vi "searchEditDevice.vi"(8 "error in (no error)":errorcluster, 11 "reference in":refnum<class "Project Panels.lvclass">=refnum) -> (0 "error out":errorcluster, 2 "saved?":bool, 3 "reference out":refnum<class "Project Panels.lvclass">)   [LabVIEW 2014, in "Project Panels.lvclass"]
uses:
  Project Panels.lvclass
  SYS/Devices Controller_llb/deviceType.ctl
  deviceState.ctl
  SYS/Devices Controller_llb/Devices Controller.lvclass
panel:
  in  "Stop Button":bool
  out "Status bar":string="Fill in the control and press Sarch Item button....."
  in  "Search Item":bool
  in  "S/N:":string
  in  "Device Type:":T1=enum."k4b2"
  out "title":string="Searching Item Panel"
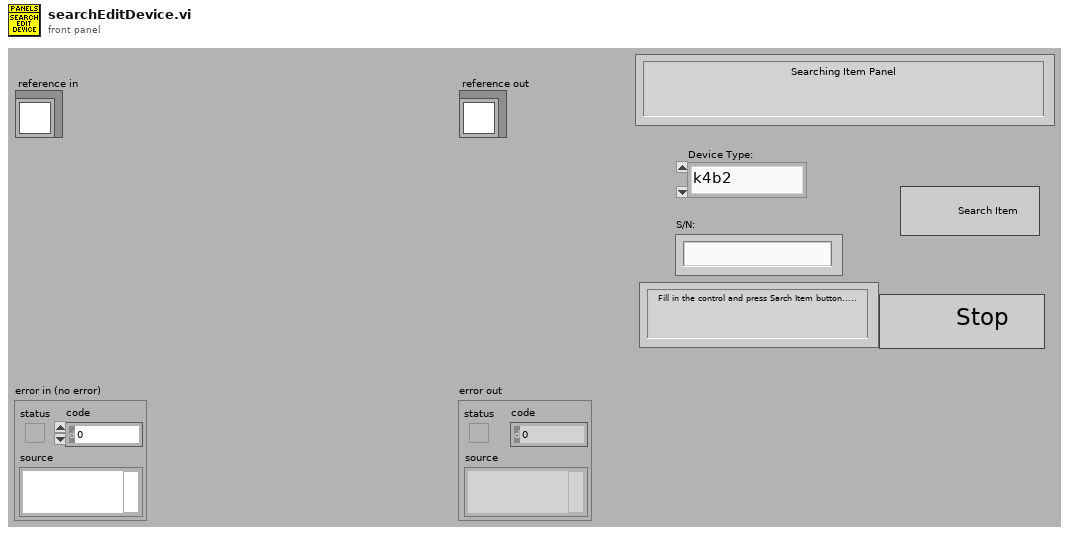
[diagram p1: front panel]
types:
  T1 = typedef "Devices Controller.lvclass/deviceType.ctl" = enum16{"k5", "k4b2", "fitmate", "cpet", "rmr", "bodyBoxPft", "bp", "pp"}
  T2 = typedef "Project Panels.lvclass/deviceState.ctl" = enum16{"check", "initiate", "waitEvent", "dataFromPDF", "getDetails", "save", "close", "stop"}
  T3 = typedef "Project Panels.lvclass/ObjectAttributesRef.ctl" = refnum<data-value>
  T4 = typedef "Project Panels.lvclass/ObjectAttributes.ctl" = cluster{"MyAttribute":dbl, "device_controller_ref":refnum<class "Devices Controller.lvclass">, "file_controller_ref":refnum<class "File Controller.lvclass">, "item_controller_ref":refnum<class "Items Controller.lvclass">, "item_tables":cluster{"checkIN":string[][], "checkOUT":string[][], "storage":string[][]}, "quickbook_table":cluster{"notes":string[][]}, "notification_controller_ref":refnum<class "Notification Controller.lvclass">, "partstracking_controller_ref":refnum<class "PartsTracking Controller.lvclass">, "product_tables":cluster{"k4b2":string[][], "fitmate":string[][], "RMR":string[][], "CPET":string[][], "BP":string[][], "PP":string[][], "k5":string[][], "bb-pft":string[][]}, "rowsColour":u32[]}
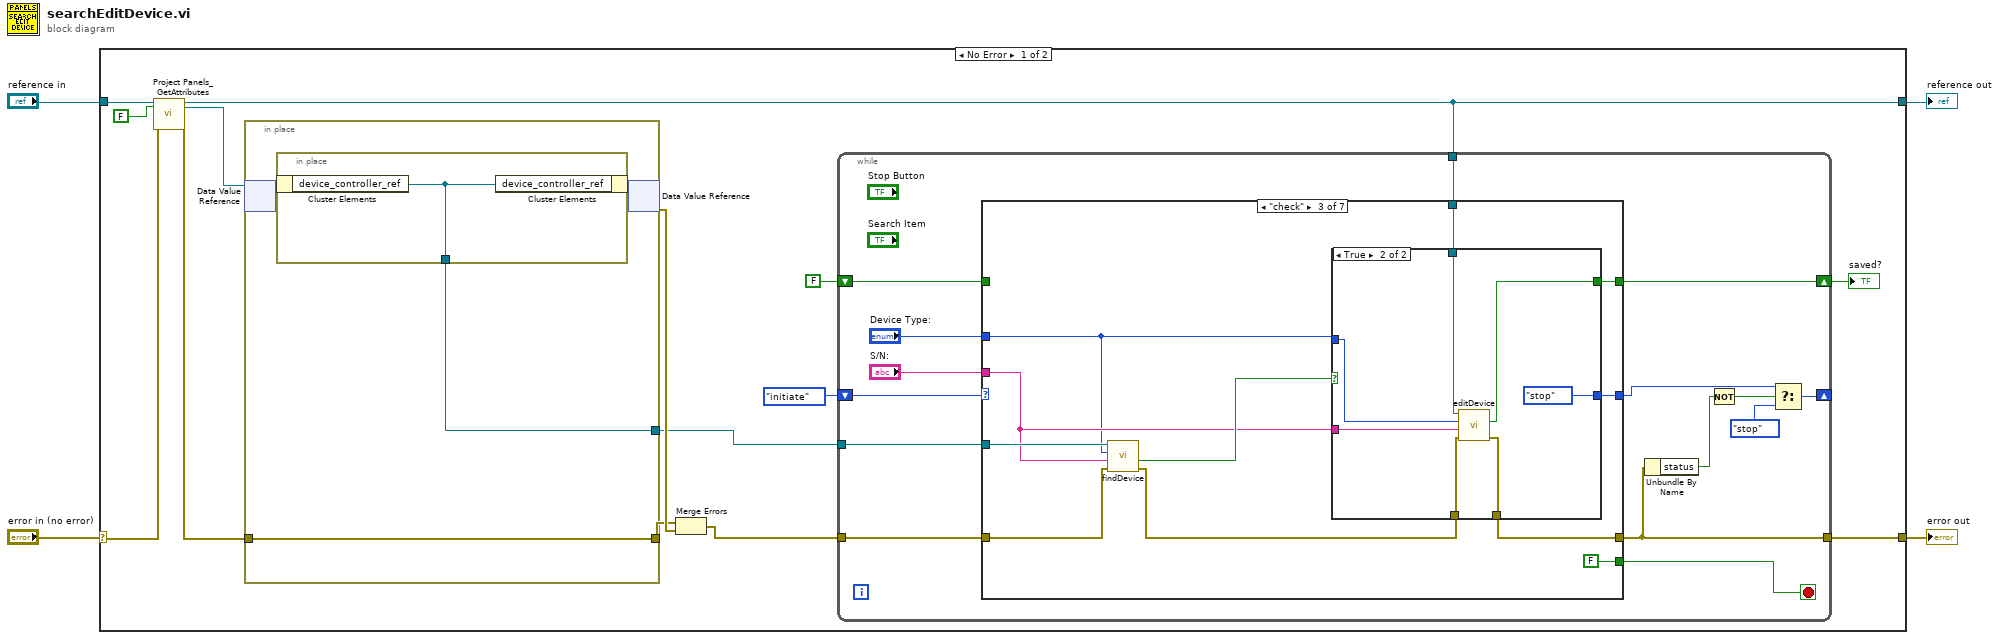
[diagram p0: block diagram]
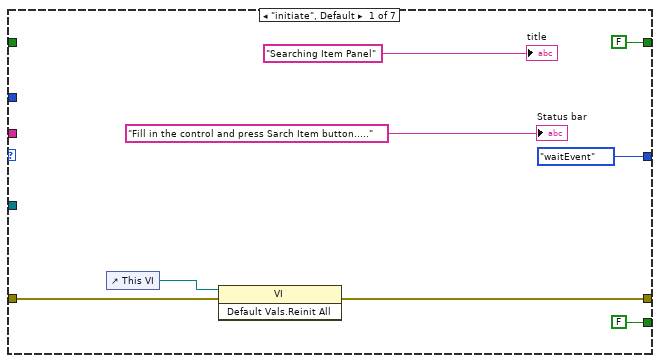
[diagram p2: hidden frame]
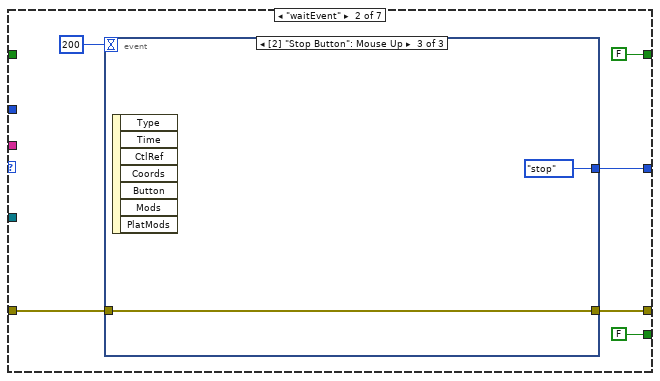
[diagram p3: hidden frame]
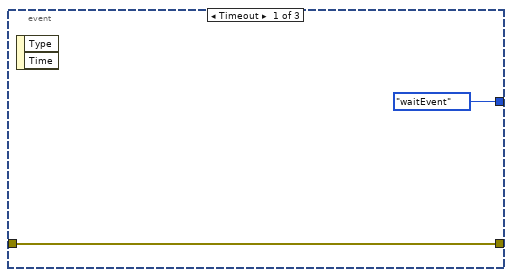
[diagram p4: hidden frame]
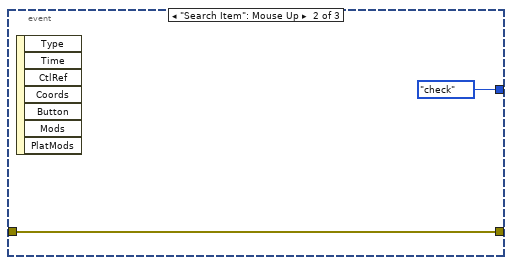
[diagram p5: hidden frame]
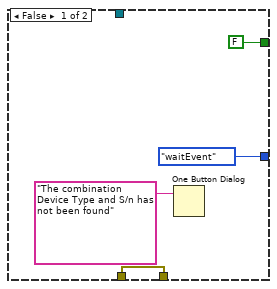
[diagram p6: hidden frame]
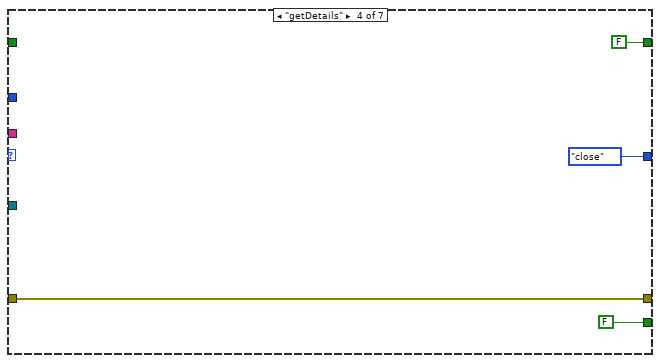
[diagram p7: hidden frame]
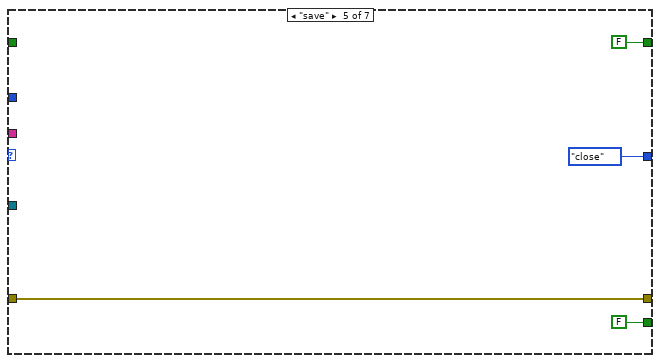
[diagram p8: hidden frame]
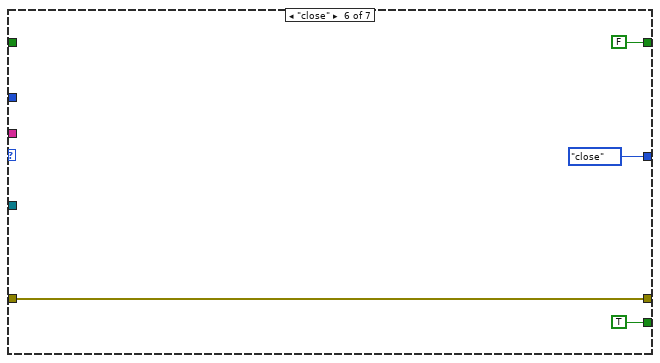
[diagram p9: hidden frame]
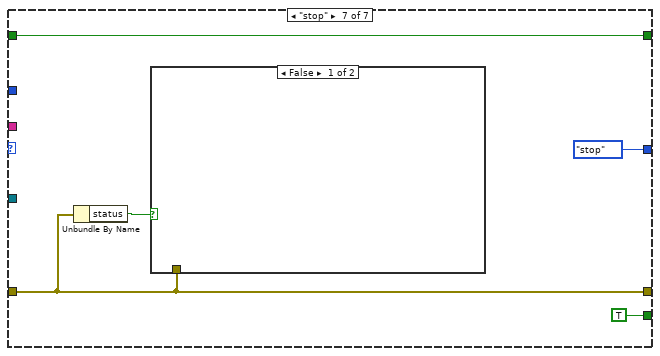
[diagram p10: hidden frame]
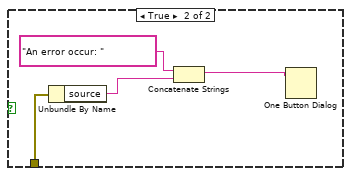
[diagram p11: hidden frame]
diagram:
  n1 = case shown="No Error" "error in (no error)" {
    selector: "error in (no error)" -> [w14 w103]
    tunnel: [w11 w103] -> w3
    tunnel: [w9 w102] -> w1
    tunnel: "reference in" -> [w16 w102]
    frame No Error {
      n2 = call "Project Panels_GetAttributes.vi"("reference in"=w16, "return data? (T)"=FALSE, "error in (no error)"=w14) -> ("reference out"=w9:refnum<class "Project Panels.lvclass">, "attributes ref"=w12:T3, "error out"=w13:errorcluster)  [unwired: 13 in, 1 out]
      n3 = in-place {
        in-place-border: w13 -> [w98]
        in-place-border: [w98] -> w17
        in-place-border: [w97] -> w5
        n4 = in-place-dvr #1(w12) -> (w99:T4)  [unwired: 1 out]
        n5 = in-place {
          in-place-border: [w101] -> w97
          n6 = in-place-cluster #2(w99) -> ("device_controller_ref"=w101:refnum<class "Devices Controller.lvclass">)
          n7 = in-place-cluster #2("device_controller_ref"=w101) -> (w100:T4)
        }
        n8 = in-place-dvr #1(w100) -> (w18:errorcluster)  [unwired: 1 out]
      }
      n9 = Merge Errors(w17, w18) -> (w6:errorcluster)
      n10 = while {
        tunnel: w6 -> [w33]
        tunnel: [w29] -> w11
        shift-right: [w30] -> _
        shift-left: deviceState."initiate" ("state") -> [w32]
        tunnel: w9 -> [w23]
        shift-right: [w21] -> w8
        shift-left: FALSE ("saved?") -> [w20]
        tunnel: w5 -> [w19]
        stop <- w22 stop-if-true
        n11 = case shown="\"check\"" w32 {
          tunnel: w33 -> [w35 w47 w59 w78 w82 w86 w89]
          tunnel: [w34 w46 w62 w78 w82 w86 w89] -> w29
          tunnel: [deviceState."waitEvent" ("state") w44 w64 deviceState."close" ("f") deviceState."close" ("f") deviceState."close" ("f") deviceState."stop" ("f")] -> w31
          tunnel: "Device Type:" -> [_ _ w54 _ _ _ _]
          tunnel: "S/N:" -> [_ _ w55 _ _ _ _]
          tunnel: w23 -> [_ _ w63 _ _ _ _]
          tunnel: [FALSE FALSE FALSE FALSE FALSE TRUE TRUE] -> w22
          tunnel: [FALSE ("saved?") FALSE ("saved?") w60 FALSE ("saved?") FALSE ("saved?") FALSE ("saved?") w88] -> w21
          tunnel: w20 -> [_ _ _ _ _ _ w88]
          tunnel: w19 -> [_ _ w57 _ _ _ _]
          frame "initiate", Default {
            n12 = control-ref of="This VI"() -> (w36:refnum<vi>)
            n13 = invoke class="VI" method="Default Vals.Reinit All"(reference=w36, error in=w35) -> (error out=w34:errorcluster)  [unwired: 1 in, 2 out]
            "title" <- "Searching Item Panel" ("title")
            "Status bar" <- "Fill in the control and press Sarch Item button....." ("Status bar")
          }
          frame "waitEvent" {
            n14 = event shown="[2] \"Stop Button\": Mouse Up" {
              selector: _ -> [_ _ _]
              dyn-events: _ -> [_ _ _]
              timeout: 200 -> [_ _ _]
              tunnel: w47 -> [w49 w51 w52]
              tunnel: [w49 w51 w52] -> w46
              tunnel: [deviceState."waitEvent" ("f") deviceState."check" ("f") deviceState."stop" ("f")] -> w44
              event Timeout {
                n15 = event-data() -> ()  [unwired: 1 in, 2 out]
              }
              event "Search Item": Mouse Up {
                n16 = event-data() -> ()  [unwired: 1 in, 7 out]
              }
              event "Stop Button": Mouse Up {
                n17 = event-data() -> ()  [unwired: 1 in, 7 out]
              }
            }
          }
          frame "check" {
            n18 = call "findDevice.vi"("error in (no error)"=w59, "S/N:"=w55, "Device Type:"=w54, "reference in"=w57) -> ("error out"=w58:errorcluster, "found!"=w56:bool)  [unwired: 4 in, 2 out]
            n19 = case shown="True" w56 {
              tunnel: [deviceState."waitEvent" ("state") deviceState."stop" ("state")] -> w64
              tunnel: w63 -> [_ w75]
              tunnel: w58 -> [w66 w74]
              tunnel: [w66 w73] -> w62
              tunnel: w55 -> [_ w72]
              tunnel: w54 -> [_ w71]
              tunnel: [FALSE ("saved?") w69] -> w60
              frame False {
                n20 = One Button Dialog(message="The combination Device Type and S/n has not been found") -> ()  [unwired: 1 in, 1 out]
              }
              frame True {
                n21 = call "editDevice.vi"("error in (no error)"=w74, "S/N IN"=w72, "Device Type In"=w71, "reference in"=w75) -> ("error out"=w73:errorcluster, "saved?"=w69:bool)  [unwired: 5 in, 1 out]
              }
            }
          }
          frame "getDetails" {
          }
          frame "save" {
          }
          frame "close" {
          }
          frame "stop" {
            n22 = Unbundle By Name(w89) -> ("status"=w90:bool)
            n23 = case shown="False" w90 {
              tunnel: w89 -> [_ w93]
              frame False {
              }
              frame True {
                n24 = Unbundle By Name(w93) -> ("source"=w94:string)
                n25 = Concatenate Strings("An error occur: " ("message"), w94) -> (w95:string)
                n26 = One Button Dialog(message=w95) -> ()  [unwired: 1 in, 1 out]
              }
            }
          }
        }
        n27 = Unbundle By Name(w29) -> ("status"=w28:bool)
        n28 = Not(x=w28) -> (.not. x?=w27:bool)
        n29 = Select(t=w31, s=w27, f=deviceState."stop") -> (s? t:f=w30:T2)
      }
      "saved?" <- w8
    }
    frame Error {
    }
  }
  "error out" <- w3
  "reference out" <- w1
